vi "niScope Set External Clock.vi"(8 "error in":errorcluster, 10 "ref. clock rate [Hz] (0: use internal clock)":dbl format="%#_13p", 11 "niScope reference in":refnum<k15>) -> (0 "error out":errorcluster, 1 "Reference Clock Rate Out":dbl, 2 "PLL Lock Status":bool, 3 "reference out":refnum<k15>, 5 "Reference Clock Source Out":string)   [LabVIEW 2018, in "niScope Virtual Digitizer.lvlib"]
doc: "Sets the clock source and clock rate for NI Scope and reads them to verify correct setting. For internal clock use 0 Hz frequency (default)."
uses:
  niScope Virtual Digitizer.lvlib
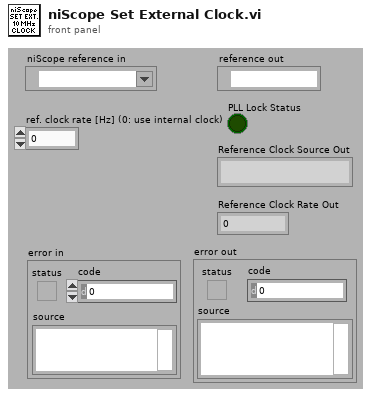
[diagram p1: front panel]
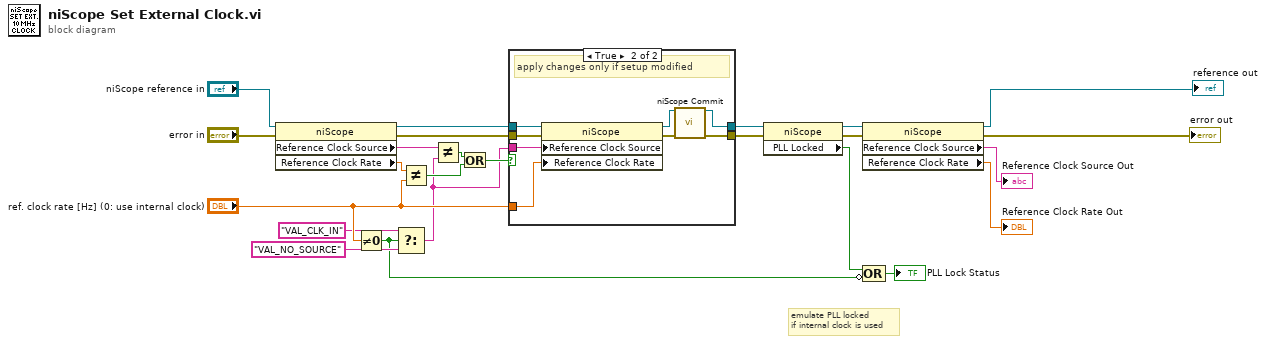
[diagram p0: block diagram]
diagram:
  # "emulate PLL locked\nif internal clock is used"
  n1 = property class="niScope"(reference="niScope reference in", error in="error in") -> (reference out=w9:refnum<k15>, error out=w14:errorcluster, "Reference Clock Source"=w5:string, "Reference Clock Rate"=w13:dbl)
  n2 = Not Equal To 0?(x="ref. clock rate [Hz] (0: use internal clock)") -> (x != 0?=w1:bool)
  n3 = Select(t="VAL_CLK_IN" ("Clocking:Reference (Input) Clock Source"), s=w1, f="VAL_NO_SOURCE" ("Clocking:Reference (Input) Clock Source")) -> (s? t:f=w4:string)
  n4 = Not Equal?(x=w13, y="ref. clock rate [Hz] (0: use internal clock)") -> (x != y?=w11:bool)
  n5 = Not Equal?(x=w5, y=w4) -> (x != y?=w12:bool)
  n6 = Or(x=w12, y=w11) -> (x .or. y?=w10:bool)
  n7 = case shown="True" w10 {
    tunnel: [w25 w32] -> w16
    tunnel: [w26 w31] -> w15
    tunnel: w9 -> [w25 w30]
    tunnel: w14 -> [w26 w29]
    tunnel: "ref. clock rate [Hz] (0: use internal clock)" -> [_ w28]
    tunnel: w4 -> [_ w27]
    frame False {
    }
    frame True {
      # "apply changes only if setup modified"
      n8 = property class="niScope"(reference=w30, error in=w29, "Reference Clock Source"=w27, "Reference Clock Rate"=w28) -> (reference out=w34:refnum<k15>, error out=w33:errorcluster)
      n9 = call <instrlib>:"niScope Commit.vi"("instrument handle"=w34, "error in"=w33) -> ("instrument handle out"=w32:refnum<k15>, "error out"=w31:errorcluster)  [unwired: 12 in]
    }
  }
  n10 = property class="niScope"(reference=w16, error in=w15) -> (reference out=w20:refnum<k15>, error out=w19:errorcluster, "PLL Locked"=w2:bool)
  n11 = property class="niScope"(reference=w20, error in=w19) -> (reference out=→"reference out":refnum<k15>, error out=→"error out":errorcluster, "Reference Clock Source"=→"Reference Clock Source Out":string, "Reference Clock Rate"=→"Reference Clock Rate Out":dbl)
  n12 = Compound Arithmetic op=OR(w2, invert w1) -> (→"PLL Lock Status":bool)
